vi "Panel.vi"(11 "Command":refnum<user-event>) -> ()   [LabVIEW 2009, in "UI Panels.lvlib" / "Panels_XControl.xctl"]
uses:
  Panels_XControl.xctl
  Typedefs/Splitter Properties.ctl
  Typedefs/Menu Event.ctl
  Controls/Panel_Command_Enum.ctl
panel:
  in  "Menu":bool
  out "Title":string
  in  "Undock":bool
  in  "Expand":bool
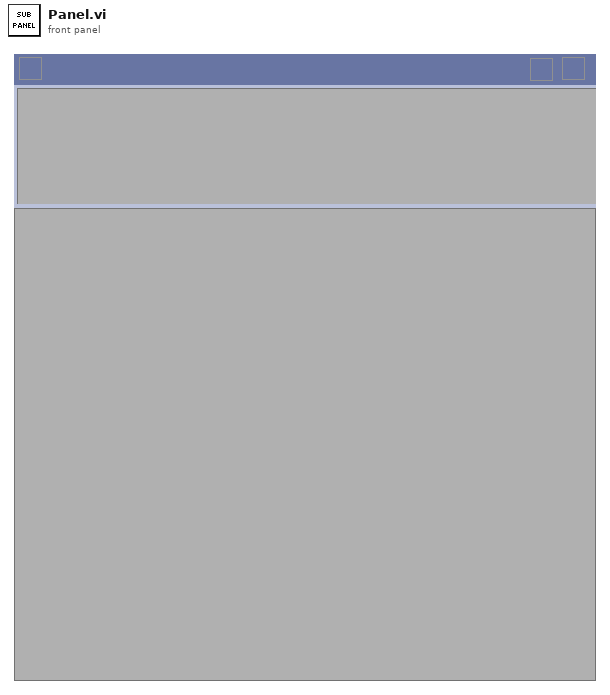
[diagram p1: front panel]
types:
  T1 = enum8{"Enabled", "Disabled", "Disabled and Grayed Out"}
  T2 = typedef "UI Panels.lvlib/Panels_XControl.xctl/Menu Event.ctl" = refnum<user-event>
  T3 = cluster{"VI Ref":refnum<vi>, "Menu Items":string[], "Menu Events":T2, "Height (Expanded)":i32, "Height (Collapsed)":i32, "Resizible":bool, "Saved Position (Upper)":i32, "Saved Position (Lower)":i32, "Position":i32, "Expanded":bool, "Title":string, "Panel Bounds":cluster{"Left":i16, "Top":i16, "Right":i16, "Bottom":i16}, "Float Panel Ref":refnum<vi>}
  T4 = typedef "UI Panels.lvlib/Panels_XControl.xctl/Splitter Properties.ctl" = cluster{"index":i32, "Height (Collapsed)":i32, "Height (Expanded)":i32, "Expanded by Default":bool, "Collapsable":bool, "Resizible":bool}
  T5 = typedef "UI Panels.lvlib/Panels_XControl.xctl/Panel_Command_Enum.ctl" = enum16{"Idle", "Remove & Stop", "Add Item", "Delete Item", "Delete All", "Insert into Subpanel", "Register Menu Events", "Update Value", "Remove from Subpanel", "Set Title", "Set Menu Items", "Insert SubPanel", "Set Splitter Position", "Set Splitter Properties", "Add Menu Items"}
  T6 = cluster{"Left":i16, "Top":i16, "Right":i16, "Bottom":i16}
  T7 = typedef "LVBoundsTypeDef.ctl" = cluster{"Width":u32, "Height":u32}
  T8 = cluster{"Left":i32, "Top":i32, "Right":u32, "Bottom":u32}
  T9 = typedef "LVRectTypeDef.ctl" = cluster{"left":i16, "top":i16, "right":i16, "bottom":i16}
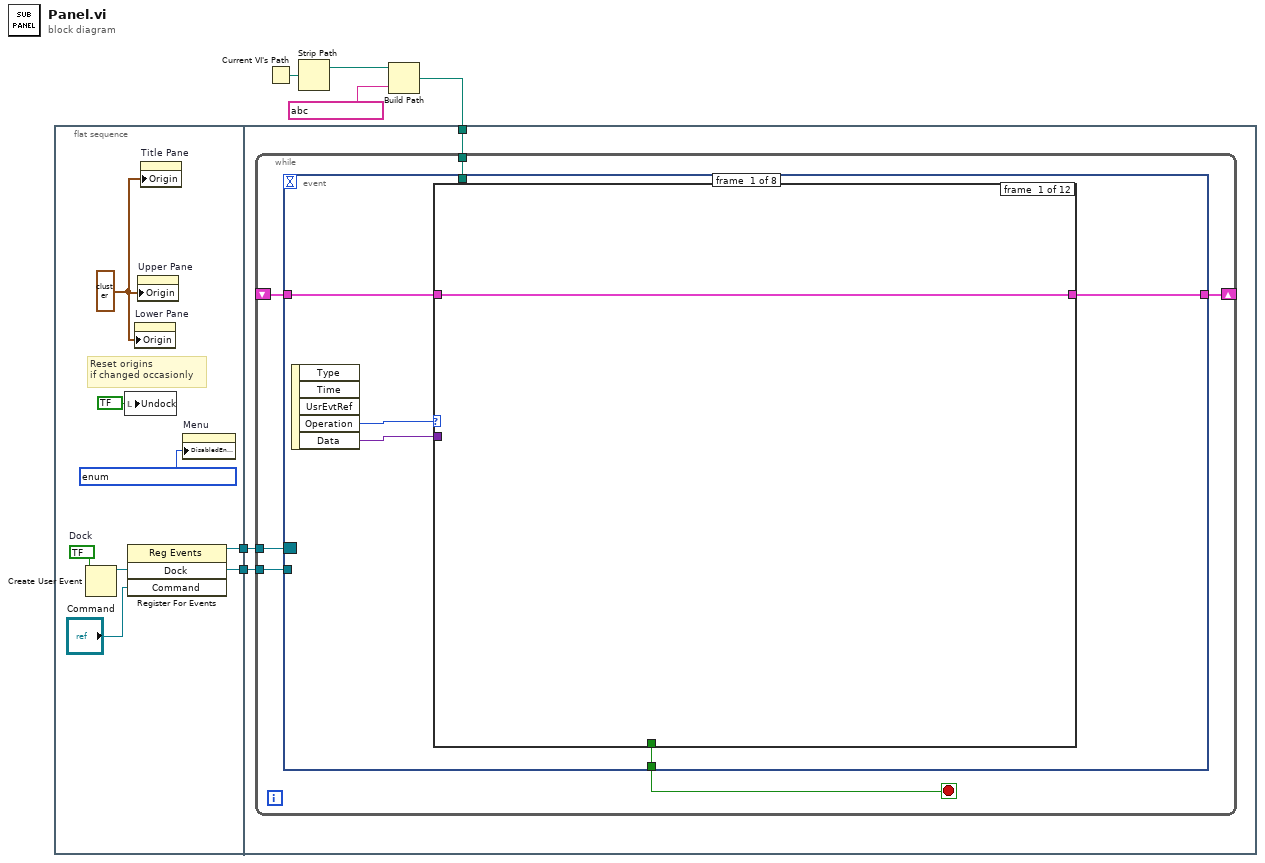
[diagram p0: block diagram]
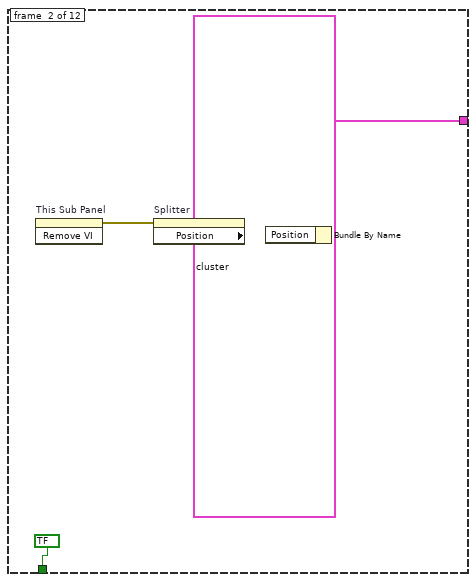
[diagram p2: hidden frame]
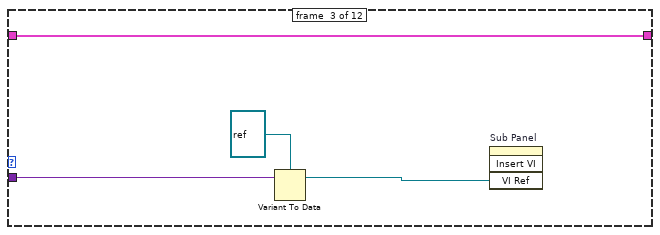
[diagram p3: hidden frame]
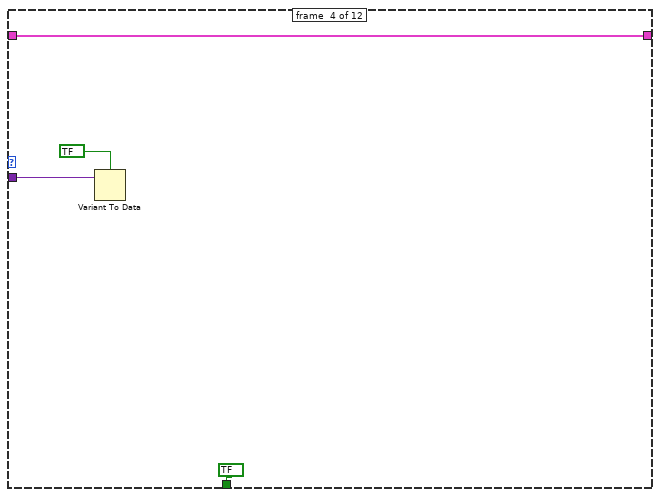
[diagram p4: hidden frame]
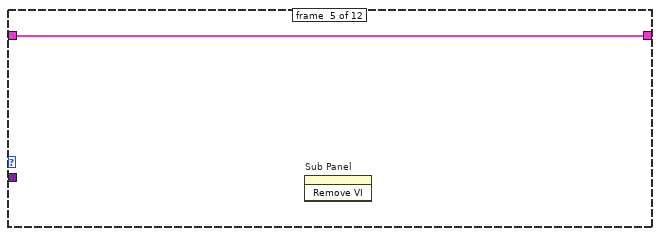
[diagram p5: hidden frame]
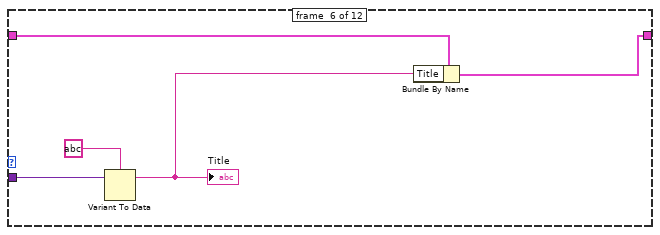
[diagram p6: hidden frame]
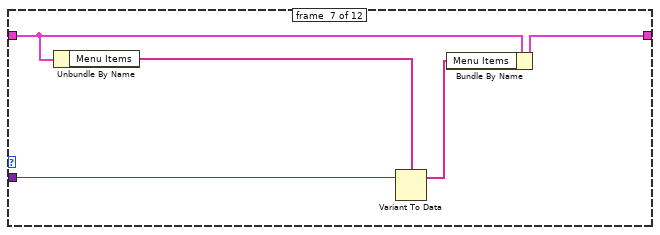
[diagram p7: hidden frame]
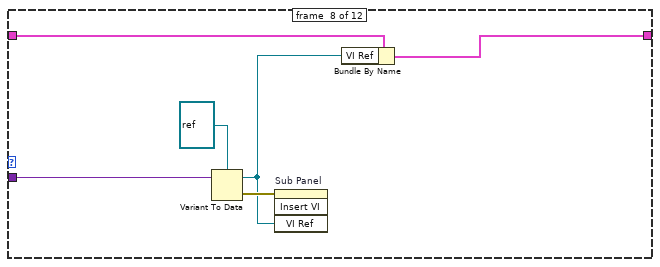
[diagram p8: hidden frame]
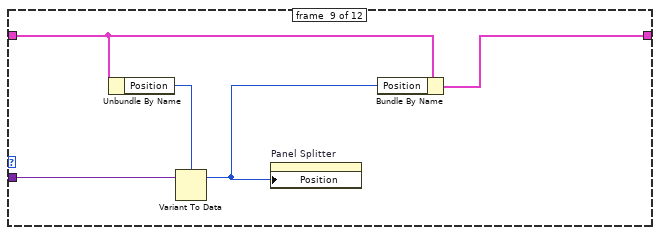
[diagram p9: hidden frame]
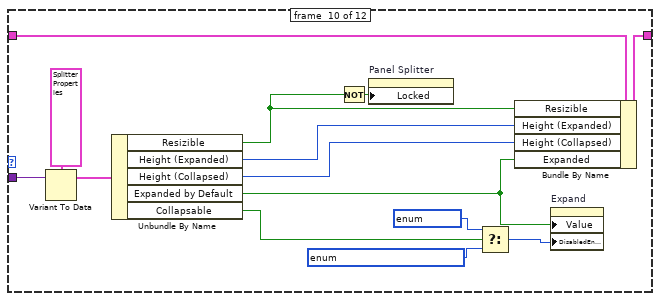
[diagram p10: hidden frame]
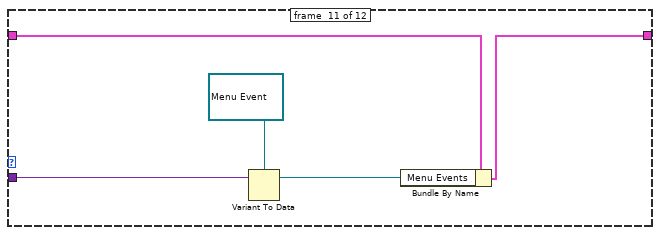
[diagram p11: hidden frame]
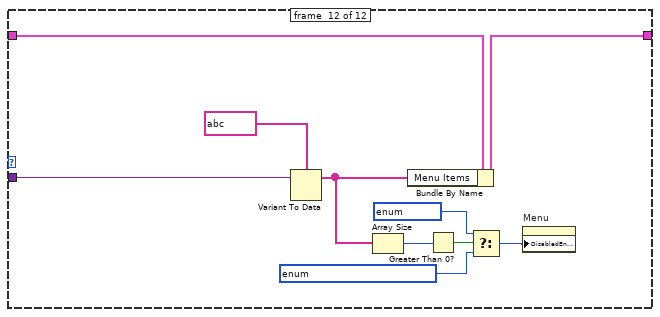
[diagram p12: hidden frame]
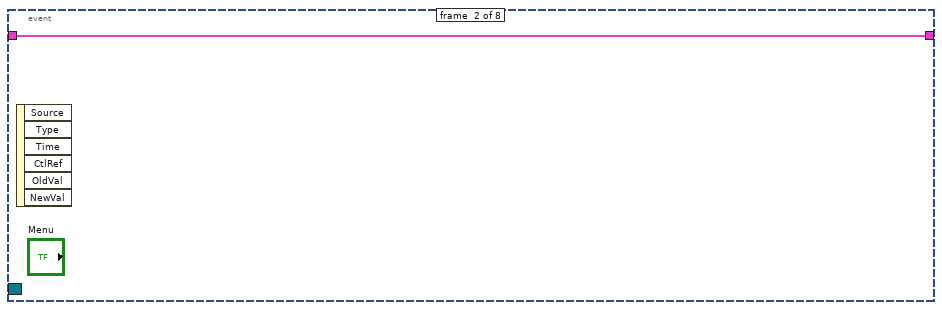
[diagram p13: hidden frame]
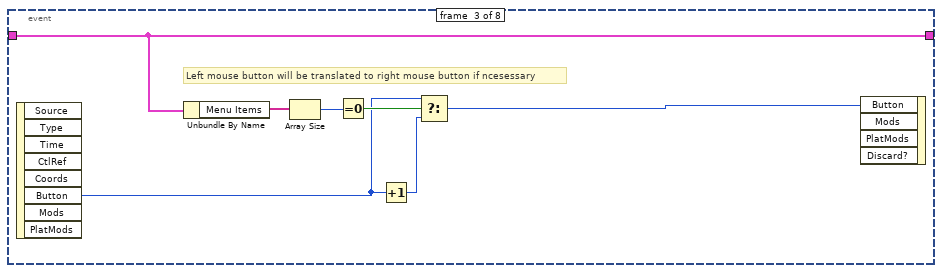
[diagram p14: hidden frame]
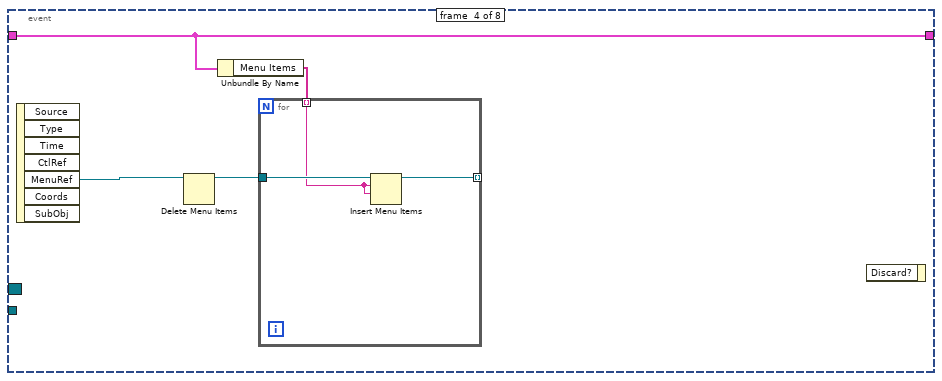
[diagram p15: hidden frame]
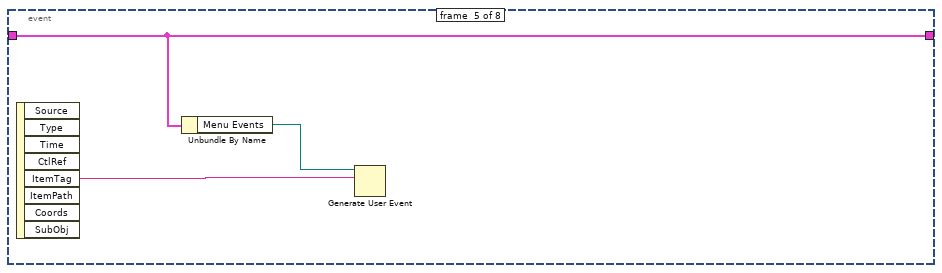
[diagram p16: hidden frame]
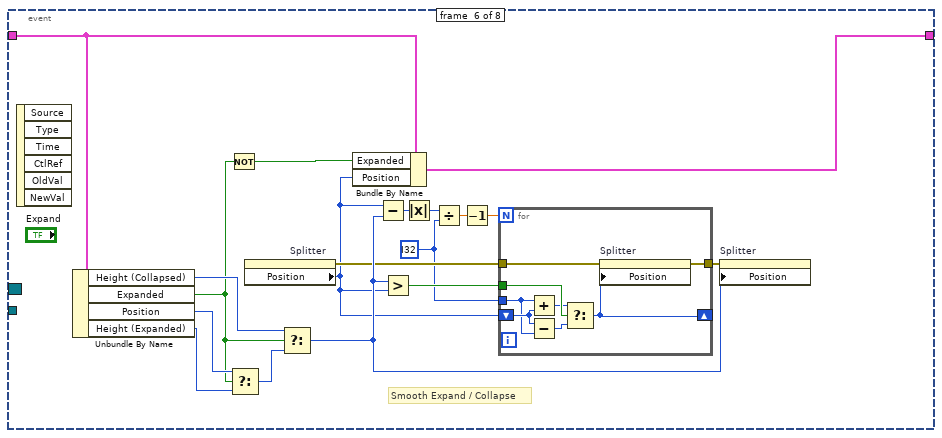
[diagram p17: hidden frame]
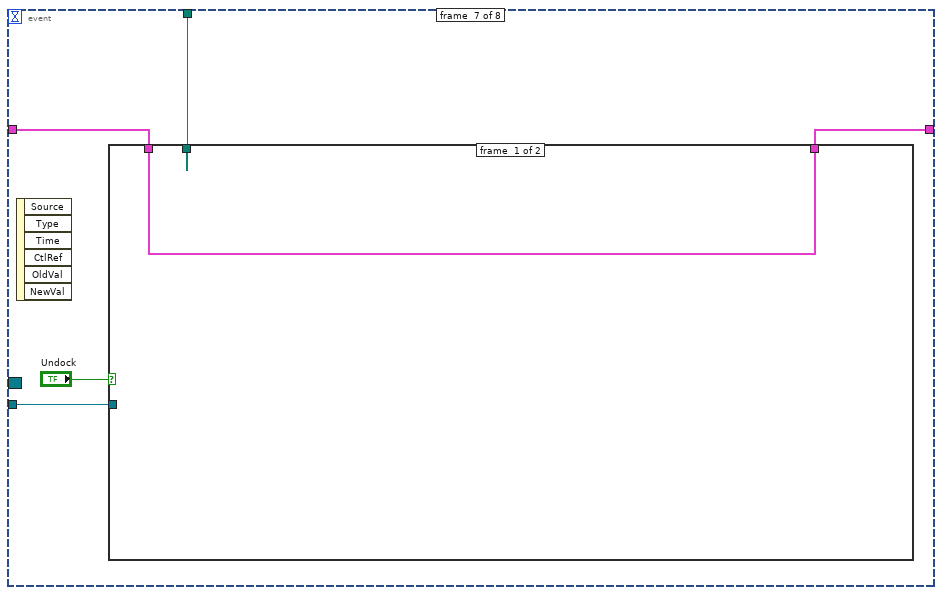
[diagram p18: hidden frame]
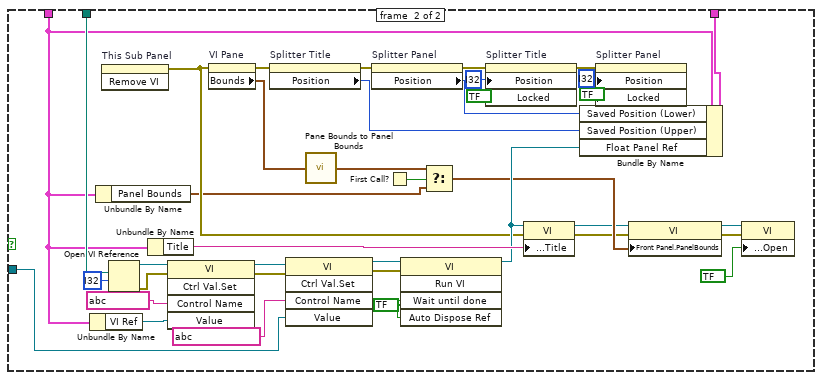
[diagram p19: hidden frame]
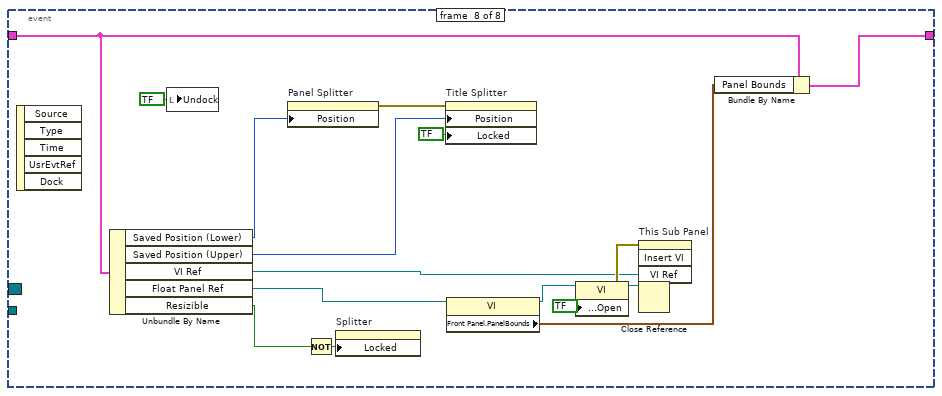
[diagram p20: hidden frame]
diagram:
  n1 = flat-sequence {
    tunnel: [w12] -> w2
    tunnel: [w11] -> w1
    tunnel: w3 -> [w16]
    tunnel: w2 -> [w15]
    tunnel: w1 -> [w14]
    frame #0 {
      w13 = bool ?  # Dock
      w10 = cluster{"Horizontal":i16, "Vertical":i16} ? ("Origin")
      # "Reset origins\nif changed occasionly"
      n2 = Create User Event(user event datatype=w13) -> (user event=w11:refnum<user-event>)  [unwired: 1 in, 1 out]
      n3 = local write "Undock"(bool ? ("Undock")) -> ()
      n4 = register-events(w11, "Command") -> (reference out=w12:refnum<event-registration>)  [unwired: 2 in, 1 out]
      n5 = property on="Lower Pane" class="Pane"("Origin"=w10) -> ()  [unwired: 2 in, 2 out]
      n6 = property on="Upper Pane" class="Pane"("Origin"=w10) -> ()  [unwired: 2 in, 2 out]
      n7 = property on="Title Pane" class="Pane"("Origin"=w10) -> ()  [unwired: 2 in, 2 out]
      n8 = property on="Menu" class="Bool"("DisabledEnum"=T1 ? ("Disabled")) -> ()  [unwired: 2 in, 2 out]
    }
    frame #1 {
      n9 = while {
        tunnel: w16 -> [w21]
        tunnel: w15 -> [w20]
        tunnel: w14 -> [w19]
        shift-right: [w18] -> _
        shift-left: _ -> [w17]
        stop <- w22 stop-if-true
        n10 = event shown="[6] \"Undock\": Value Change" {
          selector: w20 -> [_ _ _ _ _ _ _ _]
          dyn-events: _ -> [_ _ _ _ _ _ _ _]
          timeout: _ -> [_ _ _ _ _ _ _ _]
          tunnel: [w27 _ _ _ _ _ _ _] -> w22
          tunnel: w21 -> [_ _ _ _ _ _ w140 _]
          tunnel: w19 -> [_ _ _ _ _ _ w139 _]
          tunnel: [w25 w93 w100 w102 w110 w116 w137 w186] -> w18
          tunnel: w17 -> [w26 w93 w100 w102 w110 w117 w138 w187]
          event #0 {
            n11 = event-data() -> ("Operation"=w24:T5, "Data"=w23:variant)  [unwired: 4 out]
            n12 = case shown="\"Add Menu Items\"" w24 {
              tunnel: w23 -> [_ _ w37 w41 _ w47 w52 w58 w63 w77 w80 w92]
              tunnel: [_ bool ? _ bool ? _ _ _ _ _ _ _ _] -> w27
              tunnel: [w28 w31 w34 w38 w42 w44 w51 w54 w59 w71 w81 w90] -> w25
              tunnel: w26 -> [w28 _ w34 w38 w42 w45 w50 w55 w60 w72 w82 w91]
              frame #0 {
              }
              frame #1 {
                n13 = invoke on="This Sub Panel" class="SubPanel" method="Remove VI"() -> (error out=w29:errorcluster)  [unwired: 3 in, 2 out]
                n14 = property on="Splitter" class="Splitter"(error in=w29) -> ("Position"=w30:i32)  [unwired: 1 in, 2 out]
                n15 = Bundle By Name(cluster=T3 ?, "Position"=w30) -> (w31:T3)
              }
              frame #2 {
                n16 = Variant To Data(Variant=w37, type=refnum<vi> ? ("VI Refnum")) -> (data=w35:refnum<vi>)  [unwired: 1 in, 1 out]
                n17 = invoke on="Sub Panel" class="SubPnl" method="Insert VI"("VI Ref"=w35) -> ()  [unwired: 3 in, 4 out]
              }
              frame #3 {
                n18 = Variant To Data(Variant=w41, type=bool ?) -> ()  [unwired: 1 in, 2 out]
              }
              frame #4 {
                n19 = invoke on="Sub Panel" class="SubPnl" method="Remove VI"() -> ()  [unwired: 3 in, 3 out]
              }
              frame #5 {
                n20 = Variant To Data(Variant=w47, type=string ? ("Title")) -> (data=w43:string)  [unwired: 1 in, 1 out]
                "Title" <- w43
                n21 = Bundle By Name(cluster=w45, "Title"=w43) -> (w44:T3)
              }
              frame #6 {
                n22 = Unbundle By Name(w50) -> ("Menu Items"=w48:string[])
                n23 = Variant To Data(Variant=w52, type=w48) -> (data=w49:string[])  [unwired: 1 in, 1 out]
                n24 = Bundle By Name(cluster=w50, "Menu Items"=w49) -> (w51:T3)
              }
              frame #7 {
                n25 = Variant To Data(Variant=w58, type=refnum<vi> ? ("VI Refnum")) -> (error out=w56:errorcluster, data=w53:refnum<vi>)  [unwired: 1 in]
                n26 = invoke on="Sub Panel" class="SubPnl" method="Insert VI"(error in=w56, "VI Ref"=w53) -> ()  [unwired: 2 in, 4 out]
                n27 = Bundle By Name(cluster=w55, "VI Ref"=w53) -> (w54:T3)
              }
              frame #8 {
                n28 = Unbundle By Name(w60) -> ("Position"=w62:i32)
                n29 = Variant To Data(Variant=w63, type=w62) -> (data=w61:i32)  [unwired: 1 in, 1 out]
                n30 = property on="Panel Splitter" class="Splitter"("Position"=w61) -> ()  [unwired: 2 in, 2 out]
                n31 = Bundle By Name(cluster=w60, "Position"=w61) -> (w59:T3)
              }
              frame #9 {
                n32 = Variant To Data(Variant=w77, type=T4 ? ("output cluster")) -> (data=w75:T4)  [unwired: 1 in, 1 out]
                n33 = Unbundle By Name(w75) -> ("Resizible"=w65:bool, "Height (Expanded)"=w70:i32, "Height (Collapsed)"=w69:i32, "Expanded by Default"=w64:bool, "Collapsable"=w74:bool)
                n34 = Not(x=w65) -> (.not. x?=w73:bool)
                n35 = property on="Panel Splitter" class="Splitter"("Locked"=w73) -> ()  [unwired: 2 in, 2 out]
                n36 = Select(t=T1 ? ("Disabled"), s=w74, f=T1 ? ("Disabled")) -> (s? t:f=w66:T1)
                n37 = Bundle By Name(cluster=w72, "Resizible"=w65, "Height (Expanded)"=w70, "Height (Collapsed)"=w69, "Expanded"=w64) -> (w71:T3)
                n38 = property on="Expand" class="Bool (strict)"("Value"=w64, "DisabledEnum"=w66) -> ()  [unwired: 2 in, 2 out]
              }
              frame #10 {
                n39 = Variant To Data(Variant=w80, type=T2 ? ("Menu Event")) -> (data=w78:T2)  [unwired: 1 in, 1 out]
                n40 = Bundle By Name(cluster=w82, "Menu Events"=w78) -> (w81:T3)
              }
              frame #11 {
                n41 = Variant To Data(Variant=w92, type=string[] ? ("Menu")) -> (data=w83:string[])  [unwired: 1 in, 1 out]
                n42 = Array Size(array=w83) -> (size(s)=w88:i32)
                n43 = Bundle By Name(cluster=w91, "Menu Items"=w83) -> (w90:T3)
                n44 = Greater Than 0?(x=w88) -> (x > 0?=w87:bool)
                n45 = Select(t=T1 ? ("Disabled"), s=w87, f=T1 ? ("Disabled")) -> (s? t:f=w84:T1)
                n46 = property on="Menu" class="Bool"("DisabledEnum"=w84) -> ()  [unwired: 2 in, 2 out]
              }
            }
          }
          event #1 {
            n47 = event-data() -> ()  [unwired: 7 out]
          }
          event #2 {
            # "Left mouse button will be translated to right mouse button if ncesessary"
            n48 = event-data() -> ("Button"=w96:u16)  [unwired: 8 out]
            n49 = Unbundle By Name(w100) -> ("Menu Items"=w99:string[])
            n50 = Array Size(array=w99) -> (size(s)=w98:i32)
            n51 = Equal To 0?(x=w98) -> (x = 0?=w97:bool)
            n52 = Increment(x=w96) -> (x+1=w95:u16)
            n53 = Select(t=w96, s=w97, f=w95) -> (s? t:f=w94:u16)
            n54 = event-data("Button"=w94) -> ()  [unwired: 1 in, 4 out]
          }
          event #3 {
            n55 = event-data() -> ("MenuRef"=w103:refnum<k9>)  [unwired: 7 out]
            n56 = Delete Menu Items(9:w103) -> (3:w104:refnum<k9>)  [unwired: 1 in, 3 out]
            n57 = Unbundle By Name(w102) -> ("Menu Items"=w101:string[])
            n58 = for {
              tunnel: w104 -> [w107]
              tunnel: [w106] -> _ mode=indexing
              tunnel: w101 -> [w105] mode=indexing
              n59 = Insert Menu Items(7:w105, 8:w105, 9:w107) -> (3:w106:refnum<k9>)  [unwired: 1 in, 4 out]
            }
            n60 = event-data() -> ()  [unwired: 1 in, 2 out]
          }
          event #4 {
            n61 = event-data() -> ("ItemTag"=w108:string)  [unwired: 8 out]
            n62 = Unbundle By Name(w110) -> ("Menu Events"=w109:T2)
            n63 = Generate User Event(user event=w109, event data cluster=w108) -> ()  [unwired: 1 in, 2 out]
          }
          event #5 {
            w120 = i32 ? ("y")
            # "Smooth Expand / Collapse"
            n64 = event-data() -> ()  [unwired: 7 out]
            n65 = Unbundle By Name(w117) -> ("Height (Collapsed)"=w118:i32, "Expanded"=w112:bool, "Position"=w114:i32, "Height (Expanded)"=w111:i32)
            n66 = Not(x=w112) -> (.not. x?=w115:bool)
            n67 = Select(t=w114, s=w112, f=w111) -> (s? t:f=w128:i32)
            n68 = property on="Splitter" class="Splitter"() -> (error out=w123:errorcluster, "Position"=w113:i32)  [unwired: 2 in, 1 out]
            n69 = Select(t=w118, s=w112, f=w128) -> (s? t:f=w125:i32)
            n70 = Bundle By Name(cluster=w117, "Expanded"=w115, "Position"=w113) -> (w116:T3)
            n71 = Subtract(x=w113, y=w125) -> (x-y=w127:i32)
            n72 = Greater?(x=w125, y=w113) -> (0:w124:bool)
            n73 = Absolute Value(x=w127) -> (abs(x)=w126:i32)
            n74 = Divide(x=w126, y=w120) -> (x/y=w121:dbl)
            n75 = Decrement(x=w121) -> (x-1=w119:dbl)
            n76 = for {
              N: w119 -> [_]
              shift-right: [w133] -> _
              shift-left: w113 -> [w130]
              tunnel: w124 -> [w136]
              tunnel: w123 -> [w132]
              tunnel: [w131] -> w122
              tunnel: w120 -> [w129]
              n77 = Add(x=w129, y=w130) -> (x+y=w135:i32)
              n78 = Subtract(x=w130, y=w129) -> (x-y=w134:i32)
              n79 = Select(t=w135, s=w136, f=w134) -> (s? t:f=w133:i32)
              n80 = property on="Splitter" class="Splitter"(error in=w132, "Position"=w133) -> (error out=w131:errorcluster)  [unwired: 1 in, 1 out]
            }
            n81 = property on="Splitter" class="Splitter"(error in=w122, "Position"=w125) -> ()  [unwired: 1 in, 2 out]
          }
          event #6 {
            n82 = event-data() -> ()  [unwired: 7 out]
            n83 = case shown="True" "Undock" {
              tunnel: w140 -> [_ w160]
              tunnel: w139 -> [_ w173]
              tunnel: w138 -> [w142 w145]
              tunnel: [w142 w170] -> w137
              frame #0 {
              }
              frame #1 {
                w179 = bool ? ("Wait Until Done")
                n84 = Unbundle By Name(w145) -> ("VI Ref"=w171:refnum<vi>)
                n85 = Unbundle By Name(w145) -> ("Panel Bounds"=w143:T6)
                n86 = invoke on="This Sub Panel" class="SubPanel" method="Remove VI"() -> (error out=w151:errorcluster)  [unwired: 3 in, 2 out]
                n87 = Open VI Reference(vi path=w160, options=i32 ?) -> (vi reference=w175:refnum<vi>, error out=w159:errorcluster)  [unwired: 1 in, 3 out]
                n88 = Unbundle By Name(w145) -> ("Title"=w154:string)
                n89 = invoke class="VI" method="Ctrl Val.Set"(reference=w175, error in=w159, "Control Name"=string ?, "Value"=w171) -> (reference out=w176:refnum<vi>, error out=w158:errorcluster)  [unwired: 1 in, 3 out]
                n90 = property on="VI Pane" class="Pane"(error in=w151) -> (error out=w150:errorcluster, "Bounds"=w144:T7)  [unwired: 1 in, 1 out]
                n91 = property on="Splitter Title" class="Splitter"(error in=w150) -> (error out=w167:errorcluster, "Position"=w168:i32)  [unwired: 1 in, 1 out]
                n92 = invoke class="VI" method="Ctrl Val.Set"(reference=w176, error in=w158, "Control Name"=string ?, "Value"=w173) -> (reference out=w172:refnum<vi>, error out=w157:errorcluster)  [unwired: 1 in, 3 out]
                n93 = call "Pane Bounds to Panel Bounds.vi"("Pane Bounds In"=w144) -> ("Panel Bound Out"=w155:cluster{i32, i32, u32, u32})
                n94 = property on="Splitter Panel" class="Splitter"(error in=w167) -> (error out=w162:errorcluster, "Position"=w169:i32)  [unwired: 1 in, 1 out]
                n95 = First Call?() -> (First Call?: T/F=w156:bool)
                n96 = invoke class="VI" method="Run VI"(reference=w172, error in=w157, "Wait until done"=w179, "Auto Dispose Ref"=w179) -> (reference out=w153:refnum<vi>)  [unwired: 1 in, 4 out]
                n97 = Select(t=w155, s=w156, f=w143) -> (s? t:f=w152:T8)
                n98 = property on="Splitter Title" class="Splitter"(error in=w162, "Position"=i32 ? ("Splitter Position"), "Locked"=bool ? ("Splitter Position Locked")) -> (error out=w163:errorcluster)  [unwired: 1 in, 1 out]
                n99 = property class="VI"(reference=w153, error in=w151, "Front Panel.Title"=w154) -> (reference out=w149:refnum<vi>, error out=w146:errorcluster)
                n100 = Bundle By Name(cluster=w145, "Saved Position (Lower)"=w169, "Saved Position (Upper)"=w168, "Float Panel Ref"=w153) -> (w170:T3)
                n101 = property on="Splitter Panel" class="Splitter"(error in=w163, "Position"=i32 ? ("Splitter Position"), "Locked"=bool ? ("Splitter Position Locked")) -> ()  [unwired: 1 in, 2 out]
                n102 = property class="VI"(reference=w149, error in=w146, "Front Panel.PanelBounds"=w152) -> (reference out=w148:refnum<vi>, error out=w147:errorcluster)
                n103 = property class="VI"(reference=w148, error in=w147, "Front Panel.Open"=bool ? ("Front Panel Window:Open")) -> ()  [unwired: 2 out]
              }
            }
          }
          event #7 {
            n104 = event-data() -> ()  [unwired: 6 out]
            n105 = Unbundle By Name(w187) -> ("Saved Position (Lower)"=w190:i32, "Saved Position (Upper)"=w191:i32, "VI Ref"=w183:refnum<vi>, "Float Panel Ref"=w184:refnum<vi>, "Resizible"=w182:bool)
            n106 = local write "Undock"(bool ? ("Undock")) -> ()
            n107 = property on="Panel Splitter" class="Splitter"("Position"=w190) -> (error out=w192:errorcluster)  [unwired: 2 in, 1 out]
            n108 = Not(x=w182) -> (.not. x?=w189:bool)
            n109 = property on="Splitter" class="Splitter"("Locked"=w189) -> ()  [unwired: 2 in, 2 out]
            n110 = property on="Title Splitter" class="Splitter"(error in=w192, "Position"=w191, "Locked"=bool ? ("Splitter Position Locked")) -> ()  [unwired: 1 in, 2 out]
            n111 = property class="VI"(reference=w184) -> (reference out=w188:refnum<vi>, "Front Panel.PanelBounds"=w185:T9)  [unwired: 1 in, 1 out]
            n112 = property class="VI"(reference=w188, "Front Panel.Open"=bool ? ("Front Panel Window:Open")) -> (reference out=w181:refnum<vi>, error out=w195:errorcluster)  [unwired: 1 in]
            n113 = invoke on="This Sub Panel" class="SubPnl" method="Insert VI"(error in=w195, "VI Ref"=w183) -> ()  [unwired: 2 in, 4 out]
            n114 = Close Reference(reference=w181) -> ()  [unwired: 1 in, 1 out]
            n115 = Bundle By Name(cluster=w187, "Panel Bounds"=w185) -> (w186:T3)
          }
        }
      }
    }
  }
  n116 = Current VI's Path() -> (path=w5:path)
  n117 = Strip Path(path=w5) -> (stripped path=w4:path)  [unwired: 1 out]
  n118 = Build Path(base path=w4, name or relative path=string ?) -> (appended path=w3:path)
